vi "Read RingdownConfig.vi"(8 "error in (no error)":errorcluster, 11 "RingdownPlugin in":refnum<class "EraPlugin.lvclass">) -> (0 "error out":errorcluster, 2 "RingdownConfig":T1={"Config"={"p_SysOdr"=-1, "dThres"=0.0, "Preproc"={"order"=1, "f_lo"=100.0, "f_hi"=10000.0, "R_down"=-1}}, "V index"=0, "I index"=3, "PosSeq"=FALSE}, 3 "RingdownPlugin out":refnum<class "EraPlugin.lvclass">)   [LabVIEW 2017, in "AppPlugins.lvlib" / "ERAPlugin.lvclass"]
uses:
  EraPlugin.lvclass
  PublicAPI/TypeDef/RingdownConfig.ctl
  EraPlugin.lvclass/EraPlugin.ctl
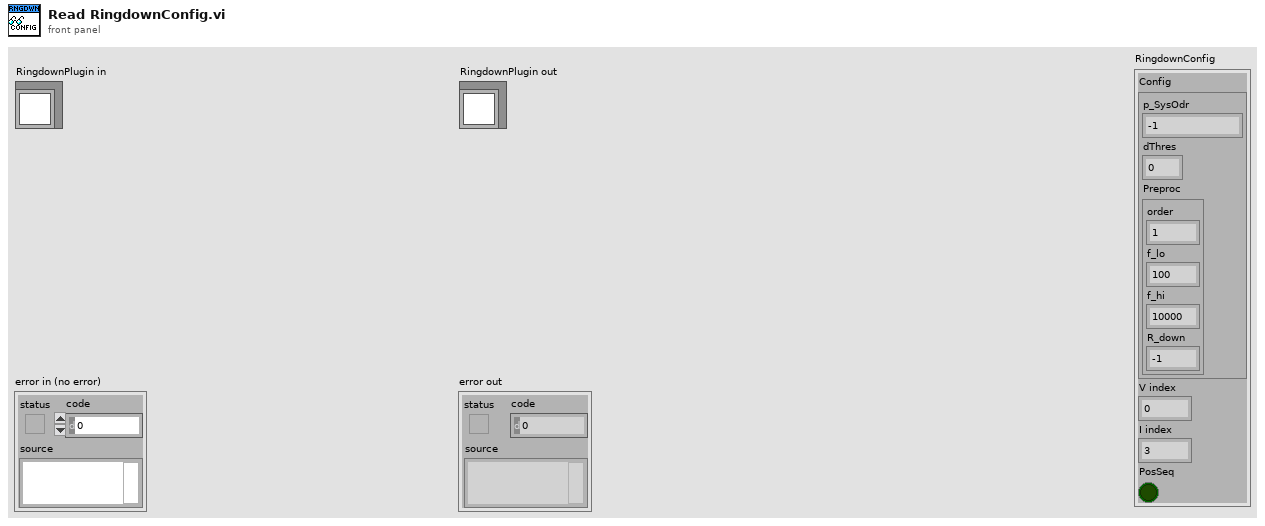
[diagram p1: front panel]
types:
  T1 = typedef "AppPlugins.lvlib/ERAPlugin.lvclass/RingdownConfig.ctl" = cluster{"Config":cluster{"p_SysOdr":i32, "dThres":dbl, "Preproc":cluster{"order":i32, "f_lo":dbl, "f_hi":dbl, "R_down":i32}}, "V index":i32, "I index":i32, "PosSeq":bool}
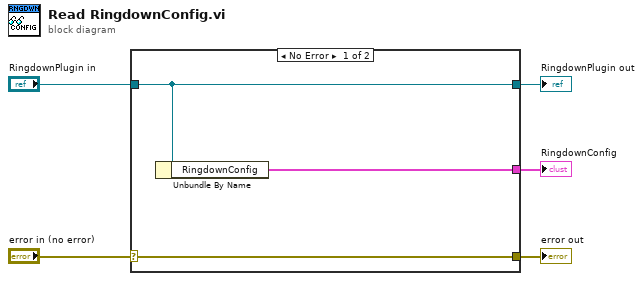
[diagram p0: block diagram]
diagram:
  n1 = case shown="No Error" "error in (no error)" {
    selector: "error in (no error)" -> [w8 w9]
    tunnel: [w8 w9] -> w4
    tunnel: [w7 w10] -> w2
    tunnel: "RingdownPlugin in" -> [w7 w10]
    tunnel: [w6 _] -> w1
    frame No Error {
      n2 = Unbundle By Name(w7) -> ("RingdownConfig"=w6:T1)
    }
    frame Error {
    }
  }
  "error out" <- w4
  "RingdownPlugin out" <- w2
  "RingdownConfig" <- w1
